vi "epics proc uniformity.vi"(8 "error in":errorcluster, 11 "CA to PROC":string) -> (0 "error out":errorcluster)   [LabVIEW 2022 SP3]
uses:
  Program Files/National Instruments/LabVIEW 2023/user.lib/calab/CaLab.lvlib
  Program Files/National Instruments/LabVIEW 2023/user.lib/calab/private/Put_String_PV.vi
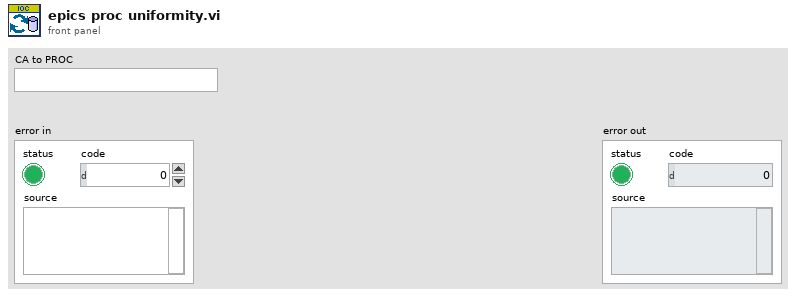
[diagram p1: front panel]
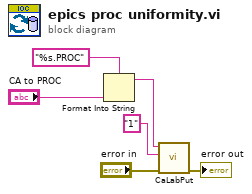
[diagram p0: block diagram]
diagram:
  n1 = Format Into String(format string="%s.PROC", "CA to PROC") -> (resulting string=w5:string)  [unwired: 2 in, 1 out]
  n2 = call-poly "CaLabPut.vi"("Error in (no error)"="error in", "Value"="1" ("format string"), "PV Name"=w5) -> ("Error out"=→"error out":errorcluster)  [unwired: 5 in, 3 out]
